vi "Compute Delta.vi"(11 "value":i32) -> (3 "delta":i32)   [LabVIEW 2017]
doc: "Uses state storage to return the absolute difference between the latest and previous values."
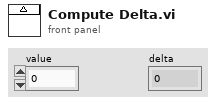
[diagram p1: front panel]
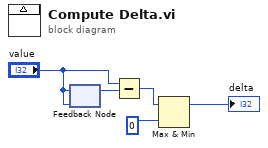
[diagram p0: block diagram]
diagram:
  n1 = feedback #1("value") -> (w4:i32)
  n2 = feedback-in #1("value") -> ()
  n3 = Subtract(x="value", y=w4) -> (x-y=w3:i32)
  n4 = Max & Min(x=w3, y=0) -> (max(x,y)=→"delta":i32)  [unwired: 1 out]
